vi "test_LoadCommandlineArgs_Version.vi"() -> (3 "Pass?":bool)   [LabVIEW 2019, in "Tests.SolutionBuilder.lvlib"]
uses:
  Tests.SolutionBuilder.lvlib
  SolutionBuilder/Community/Options.ctl
  SolutionBuilder/SolutionBuilder.lvclass
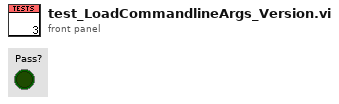
[diagram p1: front panel]
types:
  T1 = typedef "SolutionBuilder.lvlib/SolutionBuilder.lvclass/Options.ctl" = cluster{"Path":path, "Preview?":bool, "Quiet?":bool, "Log file":path, "Success file":path, "Rebuild?":bool, "Keep split projects?":bool, "Version string":string}
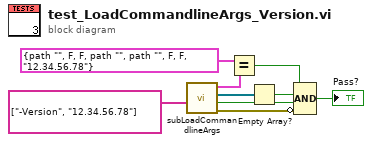
[diagram p0: block diagram]
diagram:
  n1 = call "subLoadCommandlineArgs.vi"("App.Args"=string[] ["-Version", "12.34.56.78"]) -> ("error out"=w8:errorcluster, "From command line?"=w6:bool, "Pre-built libraries"=w3:refnum<class "ProjectItem.lvclass">[], "Options"=w2:T1)  [unwired: 6 in, 1 out]
  n2 = Equal?(x=T1 {"Path"=path "", "Preview?"=FALSE, "Quiet?"=FALSE, "Log file"=path "", "Success file"=path "", "Rebuild?"=FALSE, "Keep split projects?"=FALSE, "Version string"="12.34.56.78"} ("Options"), y=w2) -> (x = y?=w5:bool)
  n3 = Empty Array?(array=w3) -> (empty?=w4:bool)
  n4 = Compound Arithmetic op=AND(w5, w4, w6, invert w8) -> (→"Pass?":bool)
